vi "ALTS-2015 Update Clamp Status.vi"(8 "error in":errorcluster, 11 "Station Cluster":T1) -> (0 "error out":errorcluster)   [LabVIEW 2013]
doc: "Copyright © 2005, Soliton Technologies.\nAll rights reserved."
uses:
  Controls/ALTS-2015 Station Cluster.ctl
  Controls/ALTS-2015 Ring Indicator Enum.ctl
  Controls/ALTS-2015 Status Ring Indicator.ctl
  Controls/ALTS-2015 Station Details.ctl
  Controls/ALTS-2015 Robot Actions.ctl
  Controls/ALTS-2015 LV2GBL Station Info Options.ctl
  Controls/ALTS-2015 Status Message Options.ctl
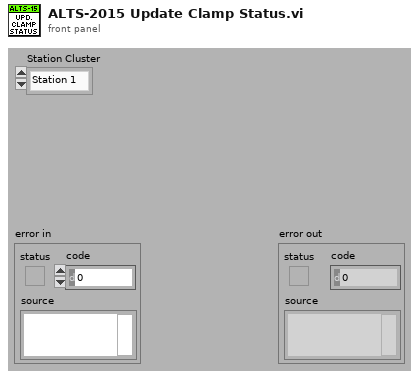
[diagram p1: front panel]
types:
  T1 = typedef "ALTS-2015 Station Cluster.ctl" = enum16{"Station 1", "Station 2", "Station 3", "Station 4"}
  T2 = typedef "ALTS-2015 Status Message Options.ctl" = enum16{"Initializing...", "Enter User Login...", "Valid Serial Number...", "Invalid Serial Number...", "Start Tag Received...", "Stop Tag Received...", "UUT Clamped...", "UUT not Clamped...", "Test Running...", "Test Complete...", "Task is assigned to robot...", "Robot is working on the task...", "Robot is ready for next task...", "Writing Result to DB...", "Idle...", "Exiting..."}
  T3 = typedef "ALTS-2015 LV2GBL Station Info Options.ctl" = enum16{"Init", "Read", "Read All", "Write Sensor ID", "Write  Work Order", "Write Serial Number", "Write Test Data", "Write Station Status", "Write Station Occupancy", "Write Station Test Type", "Write Rerun", "Write Load Decision", "Write Robot Action", "Clear All", "Clear Test Result"}
  T4 = typedef "ALTS-2015 Station Details.ctl" = cluster{"Station Number":string, "Work Order Number":string, "Sensor Name":string, "Pressure (PSI)":string, "Flow (SCCM)":string, "Test Time ":string, "Test Result":string, "Serial Number":string, "Station Status":T5, "SW assigned UUT":bool, "Rerun Count":i32, "Test Type":i32, "Load Decision":i32, "Robot Action":T6}
  T5 = typedef "ALTS-2015 Status Ring Indicator.ctl" = u16
  T6 = typedef "ALTS-2015 Robot Actions.ctl" = enum16{"Loading...", "Unloading...", "Reruning...", "No Action"}
  T7 = typedef "ALTS-2015 Ring Indicator Enum.ctl" = enum16{"Idle", "Test Running", "Unit Clamped", "Unit not Clamped", "Pass", "Fail"}
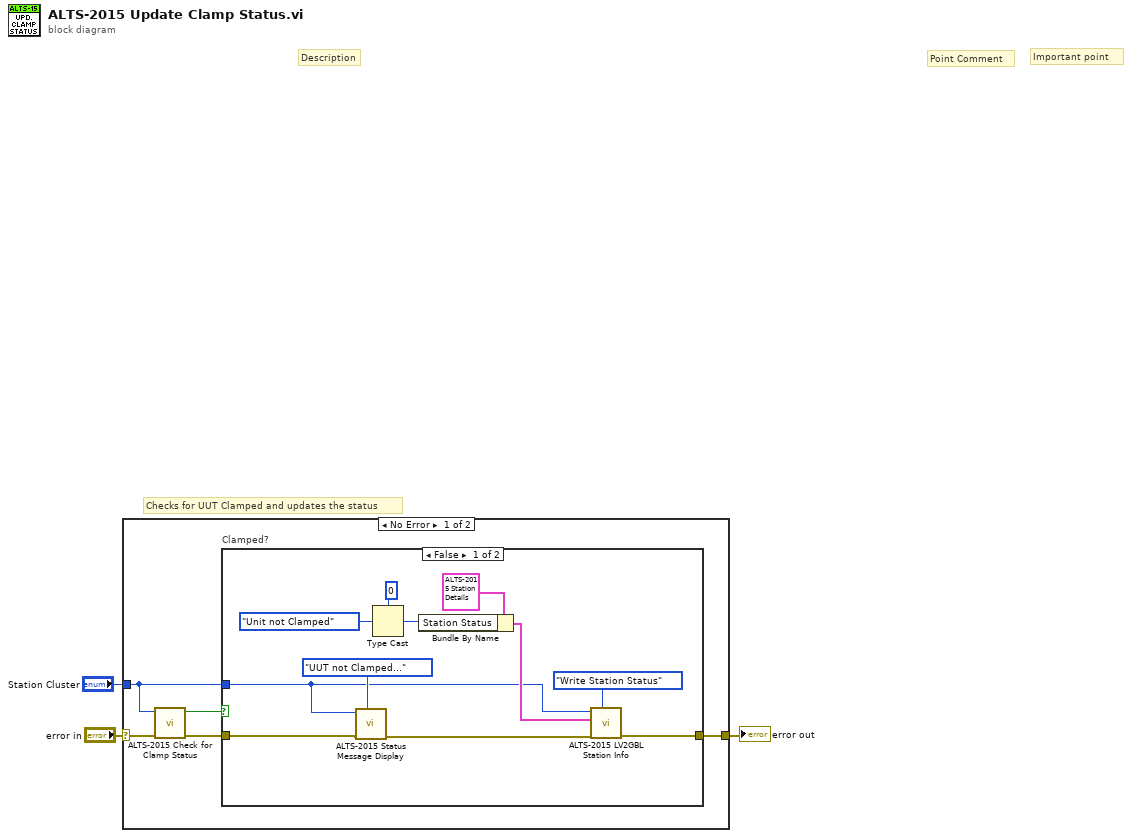
[diagram p0: block diagram]
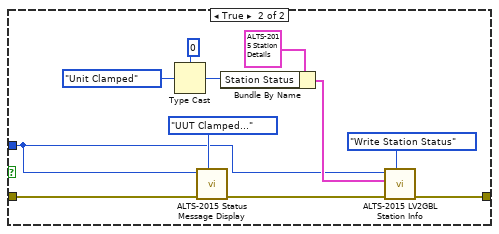
[diagram p2: hidden frame]
diagram:
  # "Checks for UUT Clamped and updates the status"
  # "Point Comment"
  # "Important point"
  # "Description"
  n1 = case shown="No Error" "error in" {
    selector: "error in" -> [w6 w30]
    tunnel: [w5 w30] -> w2
    tunnel: "Station Cluster" -> [w4 _]
    frame No Error {
      n2 = call "ALTS-2015 Check for Clamp Status .vi"("error in (no error)"=w6, "Station Cluster"=w4) -> ("error out"=w8:errorcluster, "Clamp?"=w7:bool)  [unwired: 8 in]
      n3 = case "Clamped?" shown="False" w7 {
        tunnel: w8 -> [w12 w29]
        tunnel: [w14 w21] -> w5
        tunnel: w4 -> [w9 w20]
        frame False {
          n4 = call "ALTS-2015 Status Message Display.vi"("Status Message Options"=ALTS-2015_Status_Message_Options."UUT not Clamped...", "error in (no error)"=w12, "Station Enum"=w9) -> ("error out"=w11:errorcluster)  [unwired: 7 in, 1 out]
          n5 = Type Cast(type=T5 0 ("Station Status"), x=ALTS-2015_Ring_Indicator_Enum."Unit not Clamped" ("Ring Indicator Options")) -> (*(type *) &x=w17:T5)
          n6 = Bundle By Name(cluster=T4 {"Station Number"="Station 1", "Work Order Number"="1", "Sensor Name"="Sensor 030", "Pressure (PSI)"="", "Flow (SCCM)"="", "Test Time "="", "Test Result"="", "Serial Number"="140815MOT0144", "Station Status"=2, "SW assigned UUT"=TRUE, "Rerun Count"=0, "Test Type"=3, "Load Decision"=0, "Robot Action"=enum."Loading..."} ("Station Details"), "Station Status"=w17) -> (w13:T4)
          n7 = call "ALTS-2015 LV2GBL Station Info.vi"("Options"=ALTS-2015_LV2GBL_Station_Info_Options."Write Station Status", "error in"=w11, "Station"=w13, "Station Cluster"=w9) -> ("error out"=w14:errorcluster)  [unwired: 5 in, 2 out]
        }
        frame True {
          n8 = Type Cast(type=T5 0 ("Station Status"), x=ALTS-2015_Ring_Indicator_Enum."Unit Clamped" ("Ring Indicator Options")) -> (*(type *) &x=w27:T5)
          n9 = call "ALTS-2015 Status Message Display.vi"("Status Message Options"=ALTS-2015_Status_Message_Options."UUT Clamped...", "error in (no error)"=w29, "Station Enum"=w20) -> ("error out"=w21:errorcluster)  [unwired: 7 in, 1 out]
          n10 = Bundle By Name(cluster=T4 {"Station Number"="Station 1", "Work Order Number"="1", "Sensor Name"="Sensor 030", "Pressure (PSI)"="", "Flow (SCCM)"="", "Test Time "="", "Test Result"="", "Serial Number"="140815MOT0144", "Station Status"=2, "SW assigned UUT"=TRUE, "Rerun Count"=0, "Test Type"=3, "Load Decision"=0, "Robot Action"=enum."Loading..."} ("Station Details"), "Station Status"=w27) -> (w24:T4)
          n11 = call "ALTS-2015 LV2GBL Station Info.vi"("Options"=ALTS-2015_LV2GBL_Station_Info_Options."Write Station Status", "Station"=w24, "Station Cluster"=w20) -> ()  [unwired: 6 in, 3 out]
        }
      }
    }
    frame Error {
    }
  }
  "error out" <- w2
